vi "getSourcedVoltage.vi"(7 "chn":string, 8 "error in (no error)":errorcluster, 11 "PsTti in":refnum<class "PsuTti.lvclass">) -> (0 "error out":errorcluster, 2 "Voltage":dbl, 3 "PsTti out":refnum<class "PsuTti.lvclass">)   [LabVIEW 2023, in "PsuTti.lvclass"]
doc: "Query for the actually applied voltage at the given channel."
uses:
  PsuTti.lvclass
  PsuTti.lvclass/PsuTti.ctl
  driver/Tti-Pl303Qmd.lvlib
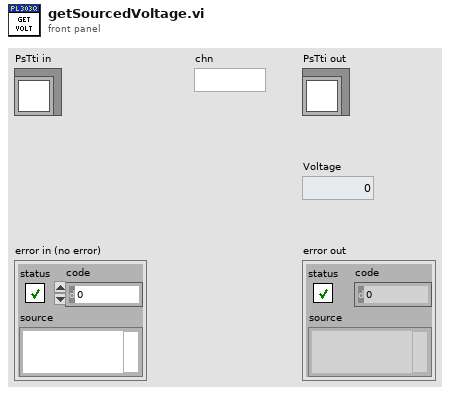
[diagram p1: front panel]
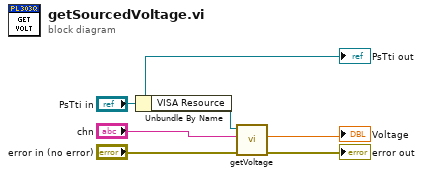
[diagram p0: block diagram]
diagram:
  n1 = Unbundle By Name("PsTti in") -> ("VISA Resource"=w2:refnum<visa-resource-name>)
  n2 = call "getVoltage.vi"("error in (no error)"="error in (no error)", "Channel Nr (1)"="chn", "VISA resource name"=w2) -> ("error out"=→"error out":errorcluster, "Voltage in Volts"=→"Voltage":dbl)  [unwired: 6 in, 1 out]
  "PsTti out" <- "PsTti in"
